vi "Hang Published Globals.vi"() -> ()   [LabVIEW 2019]
uses:
  Hang Setpoints.ctl
  Hang Operations.ctl
  <vilib>/Rock Robotics/WPI/Framework/Command Status Info.ctl
  <vilib>/Rock Robotics/WPI/Framework/Completion Status.ctl
  <vilib>/Rock Robotics/WPI/Framework/Completion Notifier.ctl
panel:
  in  "Current Command":T6
  # "Tip: The global is a good way publish state or\ninformational/debugging values.\nIt is not  advised that you put setpoint values here."
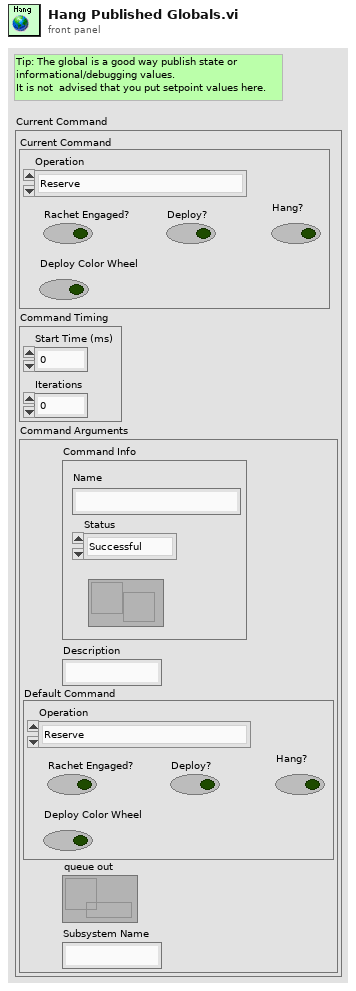
[diagram p1: front panel]
types:
  T1 = typedef "Hang Setpoints.ctl" = cluster{"Operation":T2, "Rachet Engaged?":bool, "Deploy?":bool, "Hang?":bool, "Deploy Color Wheel":bool}
  T2 = typedef "Hang Operations.ctl" = enum16{"Reserve", "Read Current", "Immediate", "Latch", "Un-Latch", "Color Wheel"}
  T3 = typedef "Command Status Info.ctl" = cluster{"Name":string, "Status":T4, "notifier out":T5}
  T4 = typedef "Completion Status.ctl" = enum16{"Successful", "Aborted", "Incomplete"}
  T5 = typedef "Completion Notifier.ctl" = refnum<notifier>
  T6 = cluster{"Current Command":T1, "Command Timing":cluster{"Start Time (ms)":u32, "Iterations":i32}, "Command Arguments":cluster{"Command Info":T3, "Description":string, "Default Command":T1, "queue out":refnum<queue>, "Subsystem Name":string}}
diagram:
